vi "Prepare Self-address.vi"(8 "error in (no error)":errorcluster, 9 "Reply to me":refnum<class "Result Reply Msg.lvclass">, 10 "Reply to":refnum<class "Result Reply Msg.lvclass">, 11 "Monitor Controller in":refnum<class "Monitor Controller.lvclass">) -> (0 "error out":errorcluster, 1 "Reply to me":refnum<class "Result Reply Msg.lvclass">, 2 "Active measurements enqueuers":refnum<class "Message Enqueuer.lvclass">[](array[class]), 3 "Monitor Controller out":refnum<class "Monitor Controller.lvclass">)   [LabVIEW 2015]
uses:
  Monitor Controller.lvclass
  Measurements/Timer Messages/Write Period Msg/Write Period Msg.lvclass
  Measure Object Messages/Result Reply Msg/Result Reply Msg.lvclass
  <vilib>/ActorFramework/Message Enqueuer/Message Enqueuer.lvclass
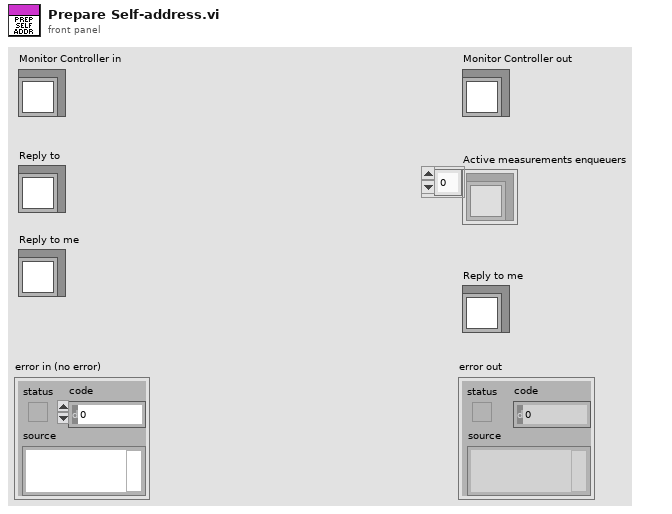
[diagram p1: front panel]
types:
  T1 = typedef "Monitor Controller Configuration.ctl" = cluster{"Period":dbl, "Repeat times":i32, "Open plot":bool}
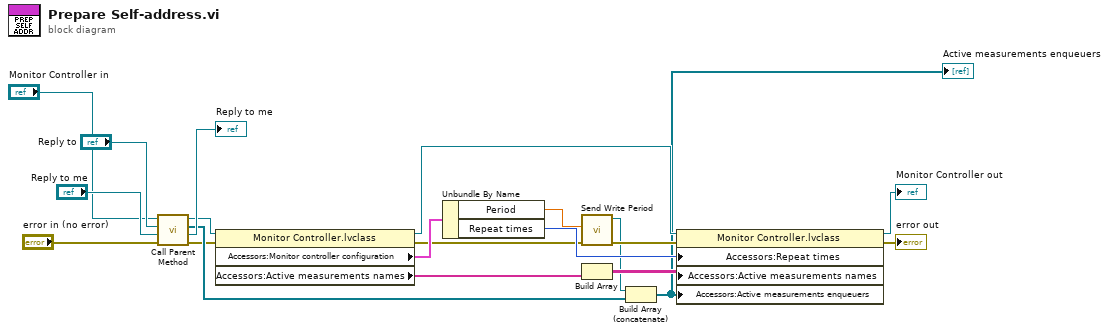
[diagram p0: block diagram]
diagram:
  n1 = call-parent "Call Parent Method"("error in (no error)"="error in (no error)", "Reply to me"="Reply to me", "Reply to"="Reply to", "Measure Controller in"="Monitor Controller in") -> ("error out"=w12:errorcluster, "Reply to me"=→"Reply to me":refnum<class "Result Reply Msg.lvclass">, "Active measurements enqueuers"=w19:refnum<class "Message Enqueuer.lvclass">[], "Measure Controller out"=w18:refnum<class "Monitor Controller.lvclass">)  [unwired: 4 in]
  n2 = property class="Monitor Controller.lvclass"(reference=w18, error in=w12) -> (reference out=w6:refnum<class "Monitor Controller.lvclass">, error out=w4:errorcluster, "Accessors:Monitor controller configuration"=w13:T1, "Accessors:Active measurements names"=w11:string[])
  n3 = Unbundle By Name(w13) -> ("Period"=w5:dbl, "Repeat times"=w9:i32)
  n4 = call "Send Write Period.vi"("error in (no error)"=w4, "Period"=w5) -> ("error out"=w3:errorcluster, "Message Enqueuer out"=w2:refnum<class "Message Enqueuer.lvclass">)  [unwired: 8 in]
  n5 = Build Array(w11) -> (w10:string[][])  [unwired: 1 in]
  n6 = Build Array (concatenate)(w2, w19) -> (w1:refnum<class "Message Enqueuer.lvclass">[])
  "Active measurements enqueuers" <- w1
  n7 = property class="Monitor Controller.lvclass"(reference=w6, error in=w3, "Accessors:Repeat times"=w9, "Accessors:Active measurements names"=w10, "Accessors:Active measurements enqueuers"=w1) -> (reference out=→"Monitor Controller out":refnum<class "Monitor Controller.lvclass">, error out=→"error out":errorcluster)
